vi "Configure Power Signals Source.vi"(6 "Voltage Channel (1: CHAN1)":i32(ring)=1 items=["CHAN1"=1, "CHAN2"=2, "CHAN3"=3, "CHAN4"=4], 7 "Voltage Name (1: Voltage 1)":i32(ring)=1 items=["Voltage 1"=1, "Voltage 2"=2], 8 "error in (no error)":errorcluster, 9 "Current Channel (2: Channel 2)":i32(ring)=2 items=["Channel 1"=1, "Channel 2"=2, "Channel 3"=3, "Channel 4"=4], 10 "Current Name (1: Current 1)":i32(ring)=1 items=["Current 1"=1, "Current 2"=2], 11 "VISA resource name":refnum<visa-resource-name>) -> (0 "error out":errorcluster, 3 "VISA resource name out":refnum<visa-resource-name>)   [LabVIEW 2010, in "Agilent 2000 3000 X-Series.lvlib"]
doc: "Specifies the current source channels and voltage source channels to be used in the power analysis."
uses:
  <instrlib>/Agilent 2000 3000 X-Series/Agilent 2000 3000 X-Series.lvlib
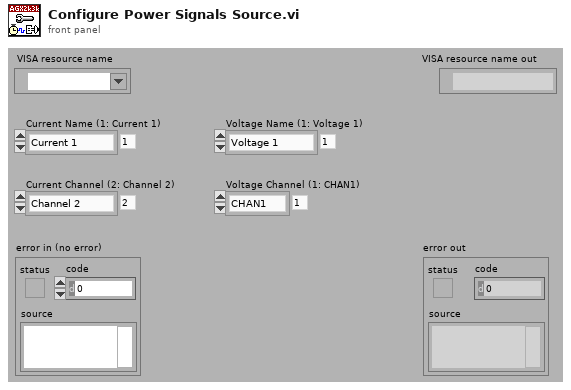
[diagram p1: front panel]
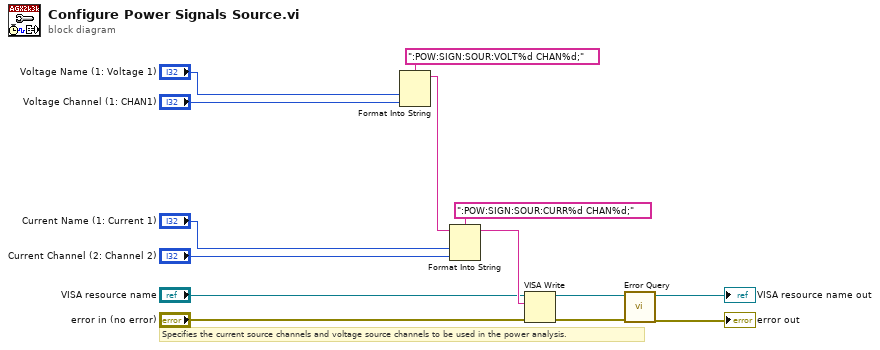
[diagram p0: block diagram]
diagram:
  # "Specifies the current source channels and voltage source channels to be used in the power analysis."
  n1 = Format Into String(format string=":POW:SIGN:SOUR:VOLT%d CHAN%d;", "Voltage Name (1: Voltage 1)", "Voltage Channel (1: CHAN1)") -> (resulting string=w13:string)  [unwired: 2 in, 1 out]
  n2 = Format Into String(format string=":POW:SIGN:SOUR:CURR%d CHAN%d;", initial string=w13, "Current Name (1: Current 1)", "Current Channel (2: Channel 2)") -> (resulting string=w11:string)  [unwired: 1 in, 1 out]
  n3 = VISA Write(VISA resource name="VISA resource name", write buffer=w11, error in (no error)="error in (no error)") -> (VISA resource name out=w8:refnum<visa-resource-name>, error out=w7:errorcluster)  [unwired: 1 out]
  n4 = call <instrlib>:"Error Query.vi"("error in (no error)"=w7, "VISA resource name"=w8) -> ("error out"=→"error out":errorcluster, "VISA resource name out"=→"VISA resource name out":refnum<visa-resource-name>)  [unwired: 8 out]
